vi "Write Save for version.vi"(8 "error in (no error)":errorcluster, 10 "Save for version":string, 11 "Control.lvclass in":refnum<class "Control.lvclass">) -> (0 "error out":errorcluster, 3 "Control.lvclass out":refnum<class "Control.lvclass">)   [LabVIEW 2012, in "Control.lvclass"]
doc: "Accessor VI for the control class"
uses:
  Control.lvclass
  Control.lvclass/Control.ctl
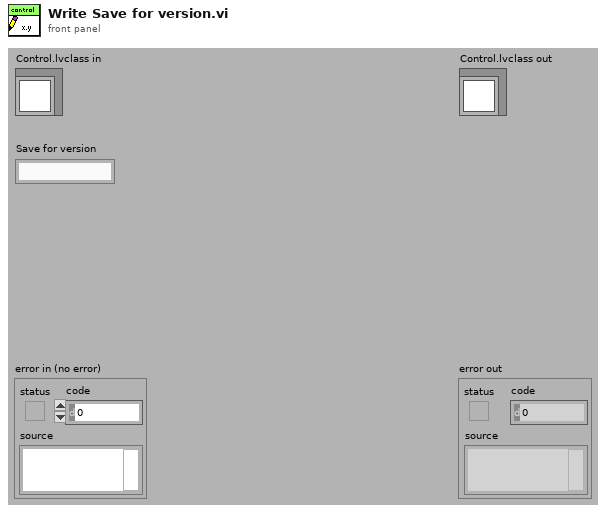
[diagram p1: front panel]
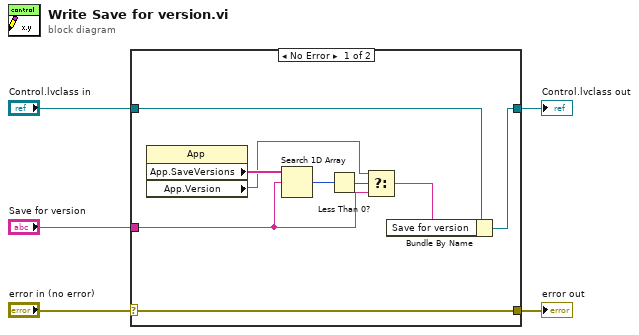
[diagram p0: block diagram]
diagram:
  n1 = case shown="No Error" "error in (no error)" {
    selector: "error in (no error)" -> [w14 w15]
    tunnel: [w14 w15] -> w4
    tunnel: [w12 w16] -> w2
    tunnel: "Control.lvclass in" -> [w13 w16]
    tunnel: "Save for version" -> [w7 _]
    frame No Error {
      n2 = property class="App"() -> ("App.SaveVersions"=w11:string[], "App.Version"=w8:string)  [unwired: 2 in, 2 out]
      n3 = Search 1D Array(1D array=w11, element=w7) -> (index of element=w10:i32)  [unwired: 1 out]
      n4 = Less Than 0?(x=w10) -> (x < 0?=w9:bool)
      n5 = Select(t=w8, s=w9, f=w7) -> (s? t:f=w6:string)
      n6 = Bundle By Name(cluster=w13, "Save for version"=w6) -> (w12:refnum<class "Control.lvclass">)
    }
    frame Error {
    }
  }
  "error out" <- w4
  "Control.lvclass out" <- w2
